vi "test performance.vi"() -> ()   [LabVIEW 2017]
uses:
  aa128119-b928-44cc-ad94-1a188039286c.vi
  aa128119-b928-44cc-ad94-1a188039286c.vi/99de0c97-112a-4c86-9094-c187659127e1.vi
  <vilib>/Utility/error.llb/Clear Errors.vi
  <vilib>/Utility/Data Type/Get Type Information.vi
  <userlib>/_NEVSTOP/Communicable State Machine(CSM)/addons/API-String-Arugments-Support/_Support/Data To SingleElementsArray_csm.vi
  <userlib>/_NEVSTOP/Communicable State Machine(CSM)/addons/API-String-Arugments-Support/_Support/Data To API String Arguments.vi
  INI-Static-Variable-Support/_Support/Parse Used Session and Name.vi
  INI-Static-Variable-Support/_Support/INI-FGV.vi
  INI-Static-Variable-Support/INI-Static-Variable-Support.lvlib
panel:
  out "x-y":u32
  out "error out":errorcluster
  in  "cluster":T1
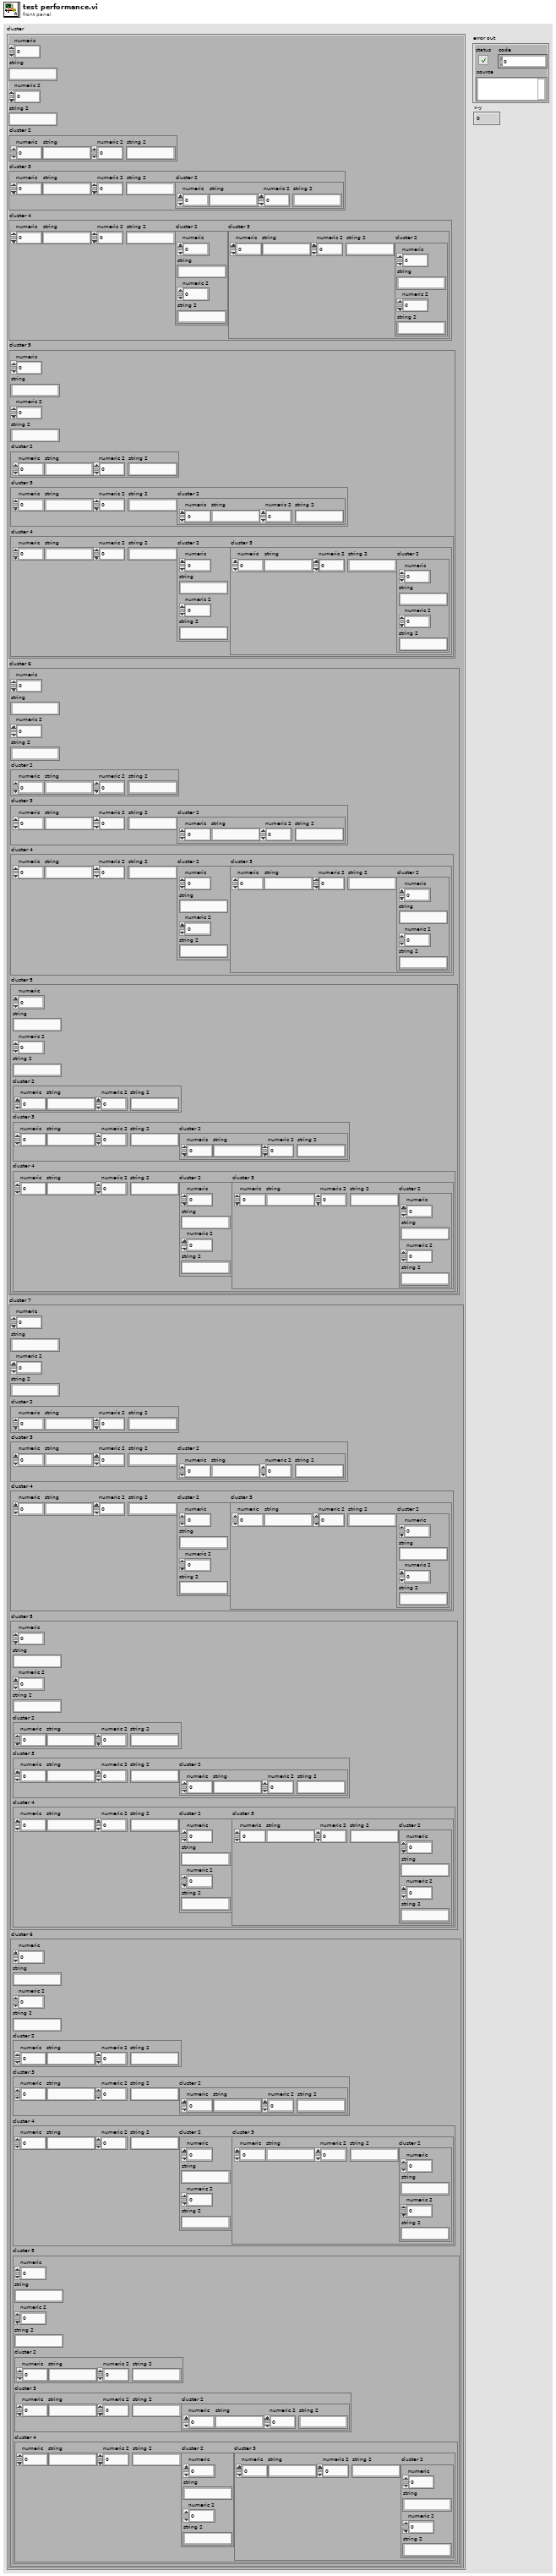
[diagram p1: front panel]
types:
  T1 = cluster{"numeric":i32, "string":string, "numeric 2":i32, "string 2":string, "cluster 2":cluster{"numeric":i32, "string":string, "numeric 2":i32, "string 2":string}, "cluster 3":cluster{"numeric":i32, "string":string, "numeric 2":i32, "string 2":string, "cluster 2":cluster{"numeric":i32, "string":string, "numeric 2":i32, "string 2":string}}, "cluster 4":cluster{"numeric":i32, "string":string, "numeric 2":i32, "string 2":string, "cluster 2":cluster{"numeric":i32, "string":string, "numeric 2":i32, "string 2":string}, "cluster 3":cluster{"numeric":i32, "string":string, "numeric 2":i32, "string 2":string, "cluster 2":cluster{"numeric":i32, "string":string, "numeric 2":i32, "string 2":string}}}, "cluster 5":cluster{"numeric":i32, "string":string, "numeric 2":i32, "string 2":string, "cluster 2":cluster{"numeric":i32, "string":string, "numeric 2":i32, "string 2":string}, "cluster 3":cluster{"numeric":i32, "string":string, "numeric 2":i32, "string 2":string, "cluster 2":cluster{"numeric":i32, "string":string, "numeric 2":i32, "string 2":string}}, "cluster 4":cluster{"numeric":i32, "string":string, "numeric 2":i32, "string 2":string, "cluster 2":cluster{"numeric":i32, "string":string, "numeric 2":i32, "string 2":string}, "cluster 3":cluster{"numeric":i32, "string":string, "numeric 2":i32, "string 2":string, "cluster 2":cluster{"numeric":i32, "string":string, "numeric 2":i32, "string 2":string}}}}, "cluster 6":cluster{"numeric":i32, "string":string, "numeric 2":i32, "string 2":string, "cluster 2":cluster{"numeric":i32, "string":string, "numeric 2":i32, "string 2":string}, "cluster 3":cluster{"numeric":i32, "string":string, "numeric 2":i32, "string 2":string, "cluster 2":cluster{"numeric":i32, "string":string, "numeric 2":i32, "string 2":string}}, "cluster 4":cluster{"numeric":i32, "string":string, "numeric 2":i32, "string 2":string, "cluster 2":cluster{"numeric":i32, "string":string, "numeric 2":i32, "string 2":string}, "cluster 3":cluster{"numeric":i32, "string":string, "numeric 2":i32, "string 2":string, "cluster 2":cluster{"numeric":i32, "string":string, "numeric 2":i32, "string 2":string}}}, "cluster 5":cluster{"numeric":i32, "string":string, "numeric 2":i32, "string 2":string, "cluster 2":cluster{"numeric":i32, "string":string, "numeric 2":i32, "string 2":string}, "cluster 3":cluster{"numeric":i32, "string":string, "numeric 2":i32, "string 2":string, "cluster 2":cluster{"numeric":i32, "string":string, "numeric 2":i32, "string 2":string}}, "cluster 4":cluster{"numeric":i32, "string":string, "numeric 2":i32, "string 2":string, "cluster 2":cluster{"numeric":i32, "string":string, "numeric 2":i32, "string 2":string}, "cluster 3":cluster{"numeric":i32, "string":string, "numeric 2":i32, "string 2":string, "cluster 2":cluster{"numeric":i32, "string":string, "numeric 2":i32, "string 2":string}}}}}, "cluster 7":cluster{"numeric":i32, "string":string, "numeric 2":i32, "string 2":string, "cluster 2":cluster{"numeric":i32, "string":string, "numeric 2":i32, "string 2":string}, "cluster 3":cluster{"numeric":i32, "string":string, "numeric 2":i32, "string 2":string, "cluster 2":cluster{"numeric":i32, "string":string, "numeric 2":i32, "string 2":string}}, "cluster 4":cluster{"numeric":i32, "string":string, "numeric 2":i32, "string 2":string, "cluster 2":cluster{"numeric":i32, "string":string, "numeric 2":i32, "string 2":string}, "cluster 3":cluster{"numeric":i32, "string":string, "numeric 2":i32, "string 2":string, "cluster 2":cluster{"numeric":i32, "string":string, "numeric 2":i32, "string 2":string}}}, "cluster 5":cluster{"numeric":i32, "string":string, "numeric 2":i32, "string 2":string, "cluster 2":cluster{"numeric":i32, "string":string, "numeric 2":i32, "string 2":string}, "cluster 3":cluster{"numeric":i32, "string":string, "numeric 2":i32, "string 2":string, "cluster 2":cluster{"numeric":i32, "string":string, "numeric 2":i32, "string 2":string}}, "cluster 4":cluster{"numeric":i32, "string":string, "numeric 2":i32, "string 2":string, "cluster 2":cluster{"numeric":i32, "string":string, "numeric 2":i32, "string 2":string}, "cluster 3":cluster{"numeric":i32, "string":string, "numeric 2":i32, "string 2":string, "cluster 2":cluster{"numeric":i32, "string":string, "numeric 2":i32, "string 2":string}}}}, "cluster 6":cluster{"numeric":i32, "string":string, "numeric 2":i32, "string 2":string, "cluster 2":cluster{"numeric":i32, "string":string, "numeric 2":i32, "string 2":string}, "cluster 3":cluster{"numeric":i32, "string":string, "numeric 2":i32, "string 2":string, "cluster 2":cluster{"numeric":i32, "string":string, "numeric 2":i32, "string 2":string}}, "cluster 4":cluster{"numeric":i32, "string":string, "numeric 2":i32, "string 2":string, "cluster 2":cluster{"numeric":i32, "string":string, "numeric 2":i32, "string 2":string}, "cluster 3":cluster{"numeric":i32, "string":string, "numeric 2":i32, "string 2":string, "cluster 2":cluster{"numeric":i32, "string":string, "numeric 2":i32, "string 2":string}}}, "cluster 5":cluster{"numeric":i32, "string":string, "numeric 2":i32, "string 2":string, "cluster 2":cluster{"numeric":i32, "string":string, "numeric 2":i32, "string 2":string}, "cluster 3":cluster{"numeric":i32, "string":string, "numeric 2":i32, "string 2":string, "cluster 2":cluster{"numeric":i32, "string":string, "numeric 2":i32, "string 2":string}}, "cluster 4":cluster{"numeric":i32, "string":string, "numeric 2":i32, "string 2":string, "cluster 2":cluster{"numeric":i32, "string":string, "numeric 2":i32, "string 2":string}, "cluster 3":cluster{"numeric":i32, "string":string, "numeric 2":i32, "string 2":string, "cluster 2":cluster{"numeric":i32, "string":string, "numeric 2":i32, "string 2":string}}}}}}}
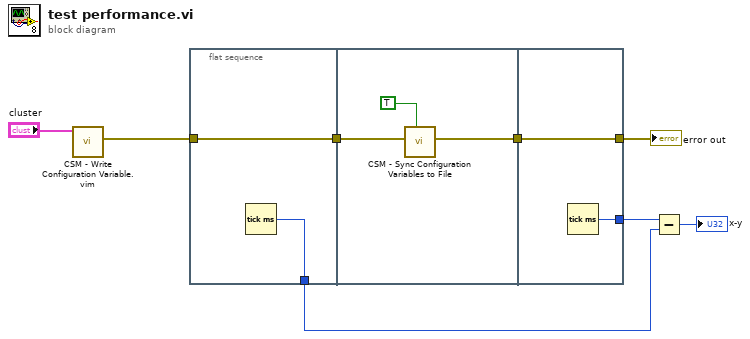
[diagram p0: block diagram]
diagram:
  n1 = call "CSM - Write Configuration Variable.vim"("Variant"="cluster") -> ("error out"=w7:errorcluster)  [unwired: 7 in, 1 out]
  n2 = flat-sequence {
    tunnel: w7 -> [w10]
    tunnel: [w10] -> w5
    tunnel: [w9] -> w2
    tunnel: w5 -> [w13]
    tunnel: [w11] -> w4
    tunnel: [w15] -> w6
    tunnel: w4 -> [w15]
    tunnel: [w14] -> w3
    frame #0 {
      n3 = Tick Count (ms)() -> (millisecond timer value=w9:u32)
    }
    frame #1 {
      n4 = call "CSM - Sync Configuration Variables to File.vi"("All Temp Variable to Default Ini(F)"=TRUE, "error in (no error)"=w13) -> ("error out"=w11:errorcluster)  [unwired: 7 in]
    }
    frame #2 {
      n5 = Tick Count (ms)() -> (millisecond timer value=w14:u32)
    }
  }
  n6 = Subtract(x=w3, y=w2) -> (x-y=→"x-y":u32)
  "error out" <- w6
